vi "Path_Manager.vi"(1 "Path_Manager_States":T1(ring), 11 "Error IN":errorcluster) -> (4 "Path":path, 15 "Error OUT":errorcluster)   [LabVIEW 2011]
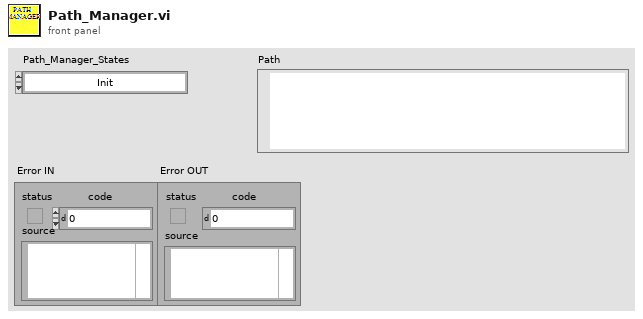
[diagram p1: front panel]
types:
  T1 = enum16{"Init", "Status", "Config Folder", "Log File Path", "Application Directory"}
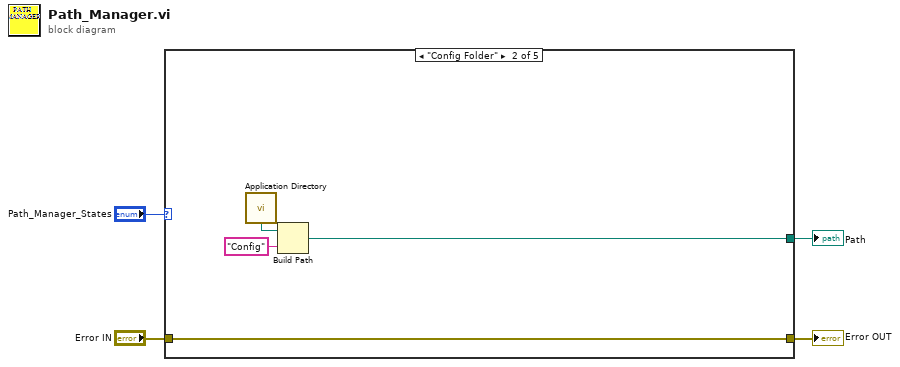
[diagram p0: block diagram]
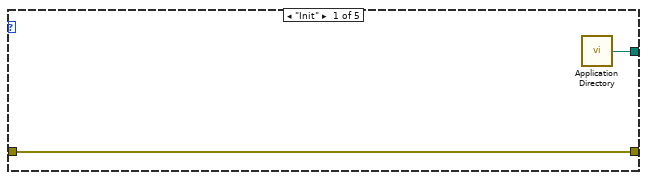
[diagram p2: hidden frame]
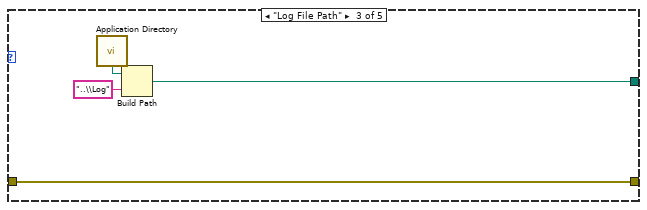
[diagram p3: hidden frame]
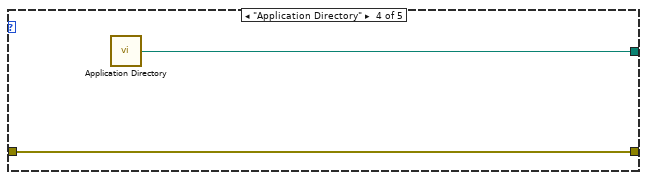
[diagram p4: hidden frame]
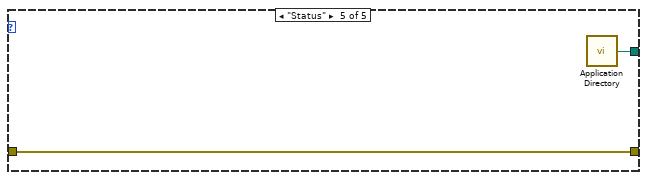
[diagram p5: hidden frame]
diagram:
  n1 = case shown="\"Config Folder\"" "Path_Manager_States" {
    tunnel: "Error IN" -> [w6 w10 w14 w16 w18]
    tunnel: [w6 w10 w14 w16 w18] -> w3
    tunnel: [w5 w7 w11 w15 w17] -> w1
    frame "Init" {
      n2 = call <vilib>:"Application Directory.vi"() -> ("Application Directory"=w5:path)
    }
    frame "Config Folder" {
      n3 = call <vilib>:"Application Directory.vi"() -> ("Application Directory"=w9:path)
      n4 = Build Path(base path=w9, name or relative path="Config") -> (appended path=w7:path)
    }
    frame "Log File Path" {
      n5 = call <vilib>:"Application Directory.vi"() -> ("Application Directory"=w13:path)
      n6 = Build Path(base path=w13, name or relative path="..\\Log") -> (appended path=w11:path)
    }
    frame "Application Directory" {
      n7 = call <vilib>:"Application Directory.vi"() -> ("Application Directory"=w15:path)
    }
    frame "Status" {
      n8 = call <vilib>:"Application Directory.vi"() -> ("Application Directory"=w17:path)
    }
  }
  "Error OUT" <- w3
  "Path" <- w1
